vi "SetEnable.vi"(10 "Enable":bool, 11 "AI in":refnum<class "AI.lvclass">) -> (3 "AI out":refnum<class "AI.lvclass">)   [LabVIEW 2019, in "AI.lvclass"]
uses:
  AI.lvclass
  AI.lvclass/AI.ctl
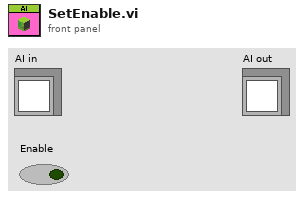
[diagram p1: front panel]
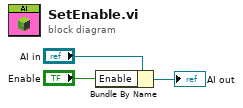
[diagram p0: block diagram]
diagram:
  n1 = Bundle By Name(cluster="AI in", "Enable"="Enable") -> (→"AI out":refnum<class "AI.lvclass">)
